vi "Magnet Enquie Message.vi"(7 "Priority Message? (F)":bool, 8 "error in (no error)":errorcluster, 9 "Message Data":variant, 10 "Message name":string, 11 "Queue in":refnum<queue>) -> (0 "error out":errorcluster, 3 "Queue out":refnum<queue>)   [LabVIEW 2017, in "Magnet module.lvlib"]
uses:
  Magnet module.lvlib
  Messenger service/Data types/Message data.ctl
  Messenger service/MessengerLib.lvlib
  ctl/MSG to magnet.ctl
  ctl/Magnet Orders.ctl
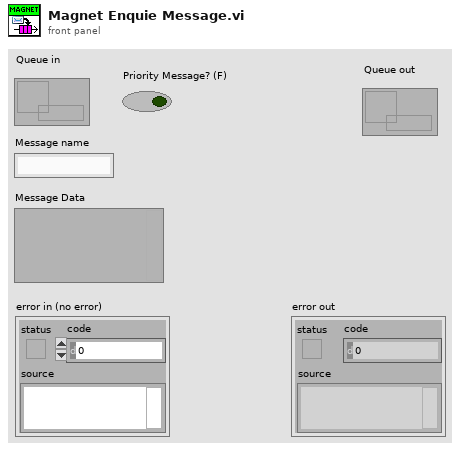
[diagram p1: front panel]
types:
  T1 = typedef "MessengerLib.lvlib/Message data.ctl" = cluster{"Name":string, "Data":variant}
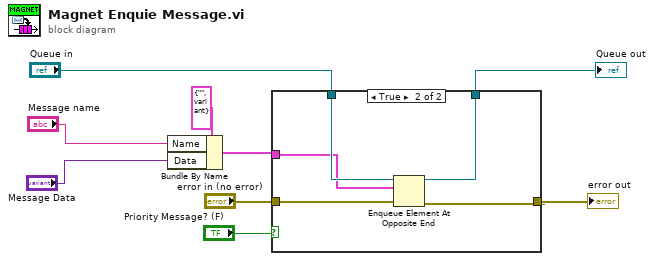
[diagram p0: block diagram]
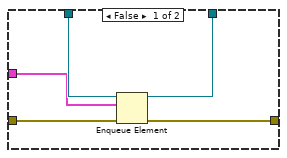
[diagram p2: hidden frame]
diagram:
  n1 = Bundle By Name(cluster=T1 {"Name"="", "Data"=variant} ("Message Cluster"), "Name"="Message name", "Data"="Message Data") -> (w1:T1)
  n2 = case shown="True" "Priority Message? (F)" {
    tunnel: "error in (no error)" -> [w13 w19]
    tunnel: [w14 w18] -> w8
    tunnel: "Queue in" -> [w12 w17]
    tunnel: w1 -> [w11 w16]
    tunnel: [w10 w15] -> w5
    frame False {
      n3 = Enqueue Element(queue=w12, element=w11, error in (no error)=w13) -> (queue out=w10:refnum<queue>, error out=w14:errorcluster)  [unwired: 1 in, 1 out]
    }
    frame True {
      n4 = Enqueue Element At Opposite End(queue=w17, element=w16, error in (no error)=w19) -> (queue out=w15:refnum<queue>, error out=w18:errorcluster)  [unwired: 1 in, 1 out]
    }
  }
  "error out" <- w8
  "Queue out" <- w5
